vi "Curvefittingtest.vi"() -> ()   [LabVIEW 2013]
uses:
  Instance           1 24Saved   Curvefittingtest .vi
  Instance           2 24Saved   Curvefittingtest .vi
  Instance           3 24Saved   Curvefittingtest .vi
panel:
  out "Array":dbl[](array[numeric])
  out "best fit":dynamicdata(graph)
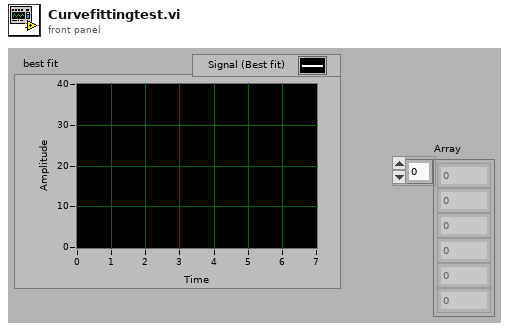
[diagram p1: front panel]
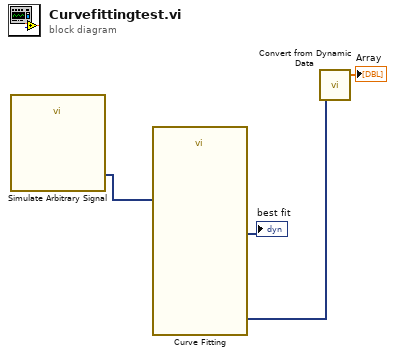
[diagram p0: block diagram]
diagram:
  n1 = call "Simulate Arbitrary Signal"() -> ("Signal"=w4:dynamicdata)  [unwired: 3 in, 8 out]
  n2 = call "Curve Fitting"("Signals"=w4) -> ("best fit"=→"best fit":dynamicdata, "polynomial coefficients"=w2:dynamicdata)  [unwired: 2 in, 7 out]
  n3 = call "Convert from Dynamic Data"("Dynamic Data Type"=w2) -> ("Array"=→"Array":dbl[])  [unwired: 3 out]
